vi "Pain-ce.vi"(0 "Lift pince":dbl, 1 "piston!!!!!!":bool) -> ()   [LabVIEW 2017]
uses:
  <vilib>/Rock Robotics/WPI/Solenoid/WPI_SolenoidValue.ctl
  <vilib>/Rock Robotics/WPI/DriverStation/WPI_DriverStationRobotMode2.ctl
  <vilib>/Rock Robotics/WPI/ThirdParty/Phoenix-LabVIEW/Motor Controller/Controls/CTRE_Phoenix_MotorControl_ControlMode.ctl
  Robot Global Data.vi
  <vilib>/Rock Robotics/Network Tables/NT Write Boolean.vi
  <vilib>/Rock Robotics/WPI/Solenoid/WPI_SolenoidSetEnum.vi
  <vilib>/Rock Robotics/WPI/ThirdParty/Phoenix-LabVIEW/Motor Controller/Get/CTRE_Phoenix_MotorController_GetQuadratureData.vi
  <vilib>/Rock Robotics/Network Tables/NT Write Number.vi
panel:
  in  "MaxHautPince":i32=188566
  out "Distance":i32
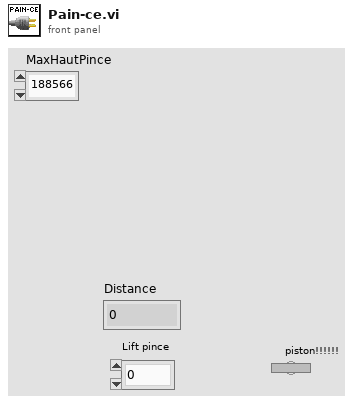
[diagram p1: front panel]
types:
  T1 = typedef "WPI_SolenoidValue.ctl" = enum16{"Off", "On", "Forward", "Reverse"}
  T2 = typedef "CTRE_Phoenix_MotorControl_ControlMode.ctl" = u16
  T3 = typedef "WPI_DriverStationRobotMode2.ctl" = enum16{"Autonomous Disabled", "Autonomous Enabled", "Teleop Disabled", "Teleop Enabled", "Disconnected", "Finish", "Test Disabled", "Test Enabled", "Emergency Stopped"}
  T4 = typedef "WPI_MotorControlDeviceRef.ctl" = cluster{"DeviceStatus":errorcluster, "Type":T5, "PWM":cluster{"PWM Channel":T6, "DeadBand":T7}, "CAN":cluster{"Device Number":u8, "SetOutput VI Ref":variant, "GetOutput VI Ref":variant, "Enable VI Ref":variant, "Disable VI Ref":variant, "Data":variant}, "Invert":bool, "DIO PWM":cluster{"PWM \"Enable\" Channel":T6, "DIOChannel":T8, "PWM Rate":dbl}}
  T5 = typedef "WPI_MotorControlType.ctl" = enum16{"PWM", "CAN", "DIO PWM"}
  T6 = typedef "FPGA_DIOPWMChannel.ctl" = enum8{"PWM 0", "PWM 1", "PWM 2", "PWM 3", "PWM 4", "PWM 5", "PWM 6", "PWM 7", "PWM 8", "PWM 9", "PWM MXP 0", "PWM MXP 1", "PWM MXP 2", "PWM MXP 3", "PWM MXP 4", "PWM MXP 5", "PWM MXP 6", "PWM MXP 7", "PWM MXP 8", "PWM MXP 9", "Invalid"}
  T7 = typedef "WPI_PWMDeadband.ctl" = cluster{"Name":string, "maxPositivePwm":i32, "minPositivePwm":i32, "centerPwm":i32, "maxNegativePwm":i32, "minNegativePwm":i32, "angularRange":u16}
  T8 = typedef "FPGA_DIOChannel.ctl" = enum8{"DIO 0", "DIO 1", "DIO 2", "DIO 3", "DIO 4", "DIO 5", "DIO 6", "DIO 7", "DIO 8", "DIO 9", "DIO MXP 0", "DIO MXP 1", "DIO MXP 2", "DIO MXP 3", "DIO MXP 4", "DIO MXP 5", "DIO MXP 6", "DIO MXP 7", "DIO MXP 8", "DIO MXP 9", "DIO MXP 10", "DIO MXP 11", "DIO MXP 12", "DIO MXP 13", "DIO MXP 14", "DIO MXP 15", "SPI Port CS1", "SPI Port CS2", "SPI Port CS3", "SPI Port MISO", "SPI Port MOSI", "Invalid"}
  T9 = typedef "WPI_SolenoidDevRef.ctl" = cluster{"DevStatus":errorcluster, "Pneumatics Control Module":u8, "Forward Solenoid Channel":T10, "Reverse Solenoid Channel":T10}
  T10 = typedef "WPI_SolenoidChannel.ctl" = enum8{"Solenoid 0", "Solenoid 1", "Solenoid 2", "Solenoid 3", "Solenoid 4", "Solenoid 5", "Solenoid 6", "Solenoid 7", "Invalid"}
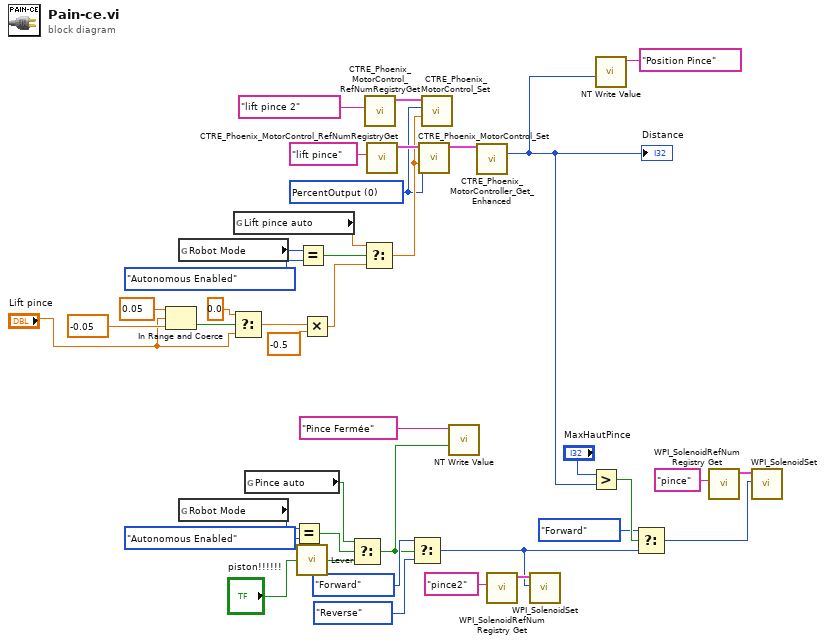
[diagram p0: block diagram]
diagram:
  w17 = T2 0 items=["PercentOutput"=0, "Position"=1, "Velocity"=2, "Current"=3, "Follower"=5, "MotionProfile"=6, "MotionMagic"=7, "MotionMagicArc"=8, "MotionProfileArc"=10, "Disabled"=15] ("Control Mode")
  n1 = In Range and Coerce(upper limit=0.05, x="Lift pince", lower limit=-0.05) -> (In Range?=w4:bool)  [unwired: 1 out]
  n2 = global read "Robot Global Data.vi" "Robot Mode"() -> (w32:T3)
  n3 = global read "Robot Global Data.vi" "Robot Mode"() -> (w35:T3)
  n4 = Select(t=0.0, s=w4, f="Lift pince") -> (s? t:f=w2:dbl)
  n5 = global read "Robot Global Data.vi" "Lift pince auto"() -> (w27:dbl)
  n6 = global read "Robot Global Data.vi" "Pince auto"() -> (w29:bool)
  n7 = Equal?(x=w35, y=WPI_DriverStationRobotMode2."Autonomous Enabled") -> (x = y?=w33:bool)
  n8 = call "Lever.vi"("Input"="piston!!!!!!") -> ("Output"=w28:bool)
  n9 = Equal?(x=w32, y=WPI_DriverStationRobotMode2."Autonomous Enabled") -> (x = y?=w30:bool)
  n10 = Multiply(x=w2, y=-0.5) -> (x*y=w14:dbl)
  n11 = Select(t=w29, s=w33, f=w28) -> (s? t:f=w24:bool)
  n12 = Select(t=w27, s=w30, f=w14) -> (s? t:f=w18:dbl)
  n13 = call <vilib>:"CTRE_Phoenix_MotorControl_RefNumRegistryGet.vi"("refnum name"="lift pince 2") -> ("PhoenixMotorControlDevRef"=w19:T4)  [unwired: 9 in, 1 out]
  n14 = call <vilib>:"CTRE_Phoenix_MotorControl_RefNumRegistryGet.vi"("refnum name"="lift pince") -> ("PhoenixMotorControlDevRef"=w26:T4)  [unwired: 9 in, 1 out]
  n15 = Select(t=WPI_SolenoidValue."Forward" ("Value"), s=w24, f=WPI_SolenoidValue."Reverse" ("Value")) -> (s? t:f=w9:T1)
  n16 = call <vilib>:"CTRE_Phoenix_MotorControl_Set.vi"("Output"=w18, "Control Mode"=w17, "PhoenixMotorControlDevRef"=w26) -> ("PhoenixMotorControlDevRef"=w22:T4)  [unwired: 7 in, 1 out]
  n17 = call <vilib>:"CTRE_Phoenix_MotorControl_Set.vi"("Output"=w18, "Control Mode"=w17, "PhoenixMotorControlDevRef"=w19) -> ()  [unwired: 7 in, 2 out]
  n18 = call-poly <vilib>:"NT Write Value.vi"("Boolean"=w24, "Name"="Pince Fermée") -> ()  [unwired: 9 in, 1 out]
  n19 = call-poly <vilib>:"CTRE_Phoenix_MotorController_Get_Enhanced.vi"("PhoenixMotorControlDevRef"=w22) -> ("Quadrature Position"=w12:i32)  [unwired: 11 in, 3 out]
  "Distance" <- w12
  n20 = call <vilib>:"WPI_SolenoidRefNum Registry Get.vi"("refnum name"="pince2") -> ("SolenoidDevRef"=w20:T9)  [unwired: 9 in, 1 out]
  n21 = call-poly <vilib>:"WPI_SolenoidSet.vi"("Value"=w9, "SolenoidDevRef"=w20) -> ()  [unwired: 8 in, 2 out]
  n22 = Greater?(x="MaxHautPince", y=w12) -> (0:w10:bool)
  n23 = call-poly <vilib>:"NT Write Value.vi"("Numeric"=w12, "Name"="Position Pince") -> ()  [unwired: 9 in, 1 out]
  n24 = Select(t=WPI_SolenoidValue."Forward", s=w10, f=w9) -> (s? t:f=w7:T1)
  n25 = call <vilib>:"WPI_SolenoidRefNum Registry Get.vi"("refnum name"="pince") -> ("SolenoidDevRef"=w38:T9)  [unwired: 9 in, 1 out]
  n26 = call-poly <vilib>:"WPI_SolenoidSet.vi"("Value"=w7, "SolenoidDevRef"=w38) -> ()  [unwired: 8 in, 2 out]
